vi "KH7008 Set Gain.vi"(4 "error in (no error)":errorcluster, 5 "Gain":u16(ring)=1 items=["1x"=1, "10x"=2, "100x"=3, "1000x"=4, "10000x"=5], 6 "Channel":u16(ring)=1 items=["Channel 1"=1, "Channel 2"=2, "Channel 3"=3, "Channel 4"=4, "Channel 5"=5, "Channel 6"=6, "Channel 7"=7, "Channel 8"=8], 7 "VISA Refnum in":refnum<visa-resource-name>="COM1") -> (0 "error out":errorcluster)   [LabVIEW 2013]
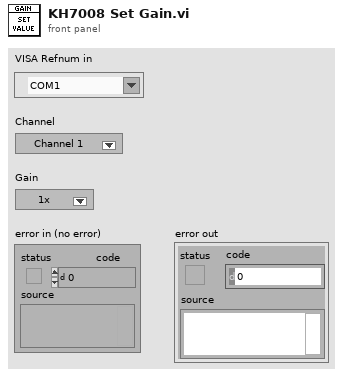
[diagram p1: front panel]
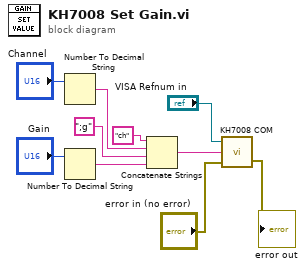
[diagram p0: block diagram]
diagram:
  n1 = Number To Decimal String(number="Channel") -> (decimal integer string=w3:string)  [unwired: 1 in]
  n2 = Number To Decimal String(number="Gain") -> (decimal integer string=w6:string)  [unwired: 1 in]
  n3 = Concatenate Strings("ch" ("string"), w3, ";g" ("string"), w6) -> (w8:string)
  n4 = call <vilib>:"KH7008 COM.vi"("error in (no error)"="error in (no error)", "Command"=w8, "VISA Refnum in"="VISA Refnum in") -> ("error out"=→"error out":errorcluster)  [unwired: 1 out]
